vi "3.1.1.4-VectorNav ParseYPR.vi"(10 "Input String":string="$VNRRG,08,+000.00,+000.00,+000.00*00") -> (0 "Roll":dbl, 1 "Pitch":dbl, 2 "Yaw":dbl)   [LabVIEW 2010]
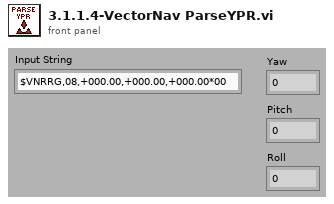
[diagram p1: front panel]
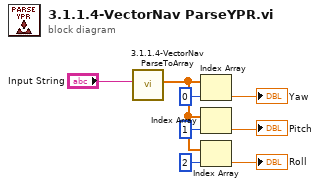
[diagram p0: block diagram]
diagram:
  n1 = call "3.1.1.4-VectorNav ParseToArray.vi"("Input String"="Input String") -> ("Output Array"=w7:dbl[])  [unwired: 10 in]
  n2 = Index Array(array=w7, index=0) -> (element=→"Yaw":dbl)
  n3 = Index Array(array=w7, index=1) -> (element=→"Pitch":dbl)
  n4 = Index Array(array=w7, index=2) -> (element=→"Roll":dbl)
